vi "ImplModelFollow_GetU_Single.vi"(9 "Index":i32, 11 "in IMPLICIT_MODEL_FOLLOWER":T1) -> (0 "Error":bool, 3 "Value":dbl)   [LabVIEW 2019, in "Trajectory_Library.lvlib"]
doc: "Returns an element of the control input vector u.\n\nInputs:\n - Implicit Model Follower -- Input data cluster\n\nOutputs:\n - Index -- Row of u.\n - U -- The control input value."
uses:
  Trajectory_Library.lvlib
  TypeDef/IMPLICIT_MODEL_FOLLOWER.ctl
  <vilib>/Analysis/Matrix/Datatypes/RealMatrix.ctl
  <vilib>/Analysis/Matrix/NI_Matrix.lvlib
panel:
  # "<States,States>"
  # "<States,Inputs>"
  # "<Inputs,1>"
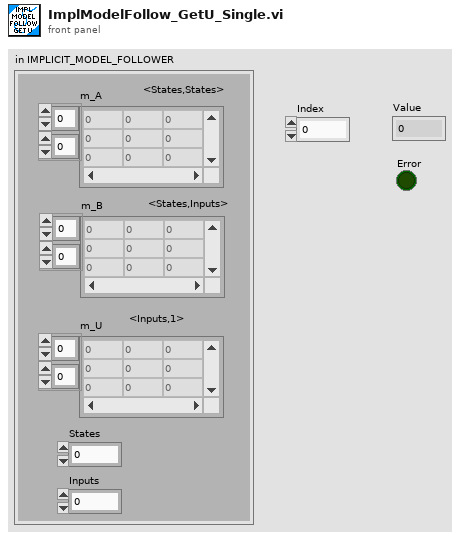
[diagram p1: front panel]
types:
  T1 = typedef "Trajectory_Library.lvlib/IMPLICIT_MODEL_FOLLOWER.ctl" = cluster{"m_A":T2, "m_B":T2, "m_U":T2, "States":i32, "Inputs":i32}
  T2 = typedef "NI_Matrix.lvlib/RealMatrix.ctl" = dbl[][]
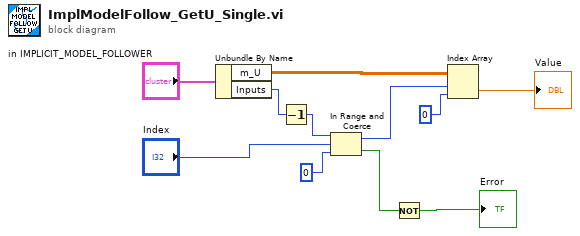
[diagram p0: block diagram]
diagram:
  n1 = Unbundle By Name("in IMPLICIT_MODEL_FOLLOWER") -> ("m_U"=w4:T2, "Inputs"=w10:i32)
  n2 = Decrement(x=w10) -> (x-1=w9:i32)
  n3 = In Range and Coerce(upper limit=w9, x="Index", lower limit=0) -> (coerced(x)=w6:i32, In Range?=w3:bool)
  n4 = Not(x=w3) -> (.not. x?=→"Error":bool)
  n5 = Index Array(array=w4, index (row)=w6, index (col)=0) -> (element=→"Value":dbl)
